vi "PII_Controller_1SDI_v01.vi"(8 "Integrator (-1)":i32, 9 "PII out (-1)":i16, 10 "Control Cavity":T1={"Lock"=FALSE, "Hold"=FALSE, "P Gain"=0, "P BS"=-5, "I Gain"=0, "I BS"=-10, "I2 G"=0, "I2 BS"=-26, "Scan Amp"=0, "Scan Off"=0, "Scan FS"=0, "SFS BS"=0, "I Max value"=10000, "I2 Max value"=10000, "Scope.Offset"=0, "Trigger Direction"=enum."either", "Scan-PII thresh"=0}, 11 "OPO A Error":i16) -> (0 "I Cavity":i32, 1 "PII out":i16, 3 "I too high?":bool)   [LabVIEW 2011]
doc: "This is a PII Controller used here to lock cavities. Pound-Drever-Hall error signals are fed in and the PII output is fed out. Designed by Seiji Armstrong, based on a design by Ben Sparkes."
uses:
  Strict Type Defs/PII individual.ctl
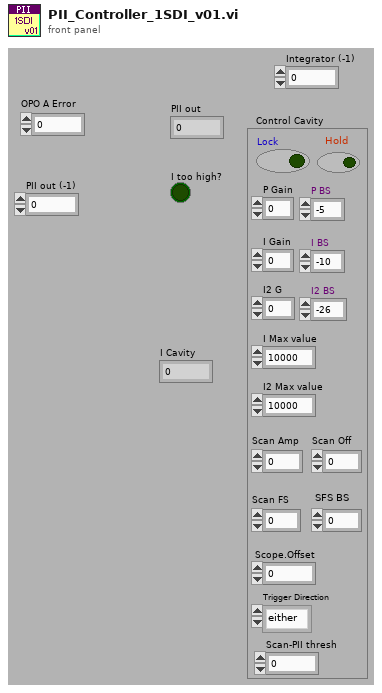
[diagram p1: front panel]
types:
  T1 = typedef "PII individual.ctl" = cluster{"Lock":bool, "Hold":bool, "P Gain":i32, "P BS":i16, "I Gain":i32, "I BS":i16, "I2 G":i32, "I2 BS":i16, "Scan Amp":i16, "Scan Off":i16, "Scan FS":u16, "SFS BS":i16, "I Max value":i32, "I2 Max value":i32, "Scope.Offset":i16, "Trigger Direction":enum8{"either", "minus-plus", "plus-minus"}, "Scan-PII thresh":i16}
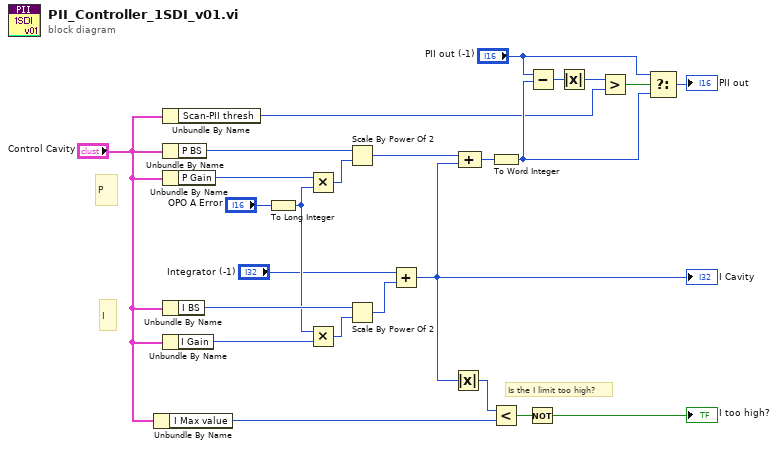
[diagram p0: block diagram]
diagram:
  # "Is the I limit too high?"
  # "P"
  # "I"
  n1 = Unbundle By Name("Control Cavity") -> ("I Max value"=w16:i32)
  n2 = Unbundle By Name("Control Cavity") -> ("Scan-PII thresh"=w6:i16)
  n3 = Unbundle By Name("Control Cavity") -> ("P BS"=w23:i16)
  n4 = Unbundle By Name("Control Cavity") -> ("P Gain"=w18:i32)
  n5 = Unbundle By Name("Control Cavity") -> ("I BS"=w21:i16)
  n6 = Unbundle By Name("Control Cavity") -> ("I Gain"=w22:i32)
  n7 = To Long Integer(number="OPO A Error") -> (32bit integer=w4:i32)
  n8 = Multiply(x=w18, y=w4) -> (x*y=w24:i32)
  n9 = Multiply(x=w4, y=w22) -> (x*y=w20:i32)
  n10 = Scale By Power Of 2(n=w23, x=w24) -> (x*2^n=w19:i32)
  n11 = Scale By Power Of 2(n=w21, x=w20) -> (x*2^n=w2:i32)
  n12 = Add(x="Integrator (-1)", y=w2) -> (x+y=w1:i32)
  "I Cavity" <- w1
  n13 = Absolute Value(x=w1) -> (abs(x)=w25:i32)
  n14 = Compound Arithmetic op=ADD(w19, w1) -> (w13:i32)
  n15 = To Word Integer(number=w13) -> (16bit integer=w10:i16)
  n16 = Less?(x=w25, y=w16) -> (x < y?=w5:bool)
  n17 = Not(x=w5) -> (.not. x?=→"I too high?":bool)
  n18 = Subtract(x="PII out (-1)", y=w10) -> (x-y=w12:i16)
  n19 = Absolute Value(x=w12) -> (abs(x)=w7:i16)
  n20 = Greater?(x=w7, y=w6) -> (0:w11:bool)
  n21 = Select(t="PII out (-1)", s=w11, f=w10) -> (s? t:f=→"PII out":i16)
